vi "ZE_Recorder_CheckChannelDuplicates.vi"(8 "error in":errorcluster, 11 "Channel Array":T1 {"Terminal" items=["Default"=-1, "RSE"=10083, "NRSE"=10078, "Differential"=10106, "Pseudodifferential"=12529]}) -> (0 "error out":errorcluster, 1 "Multi Device":bool, 2 "No of channels":i16, 3 "Channel Array out":T1 caption="Channel Array" {"Terminal" items=["Default"=-1, "RSE"=10083, "NRSE"=10078, "Differential"=10106, "Pseudodifferential"=12529]})   [LabVIEW 2025, in "ZE_Recorder.lvlib"]
doc: "ZE_Recorder_CheckChannelDuplicates.vi\n----------------------------------------------\nChecks if all channels are valid and that no duplicates exist. Returns the number of valid channels or -1 in case of error.\n\nInputs:\n---------------------\n- error in : Cluster; \n- Channel Array : 1DArrayOfCluster; \n\nOutputs:\n---------------------\n- error out : Cluster; \n- No of channels : I16; \n\n----------------------------------------------\n24.08.2016\nZühlke Engineering AG\nCH-8952 Schlieren\nwww.zuehlke.com"
uses:
  ZE_Recorder.lvlib
  ZE_Recorder_ChannelCluster.ctl
  ChannelCluster.ctl
  ZE_Recorder_Units.ctl
  Temperature.ctl
panel:
  # "Connector Pane"
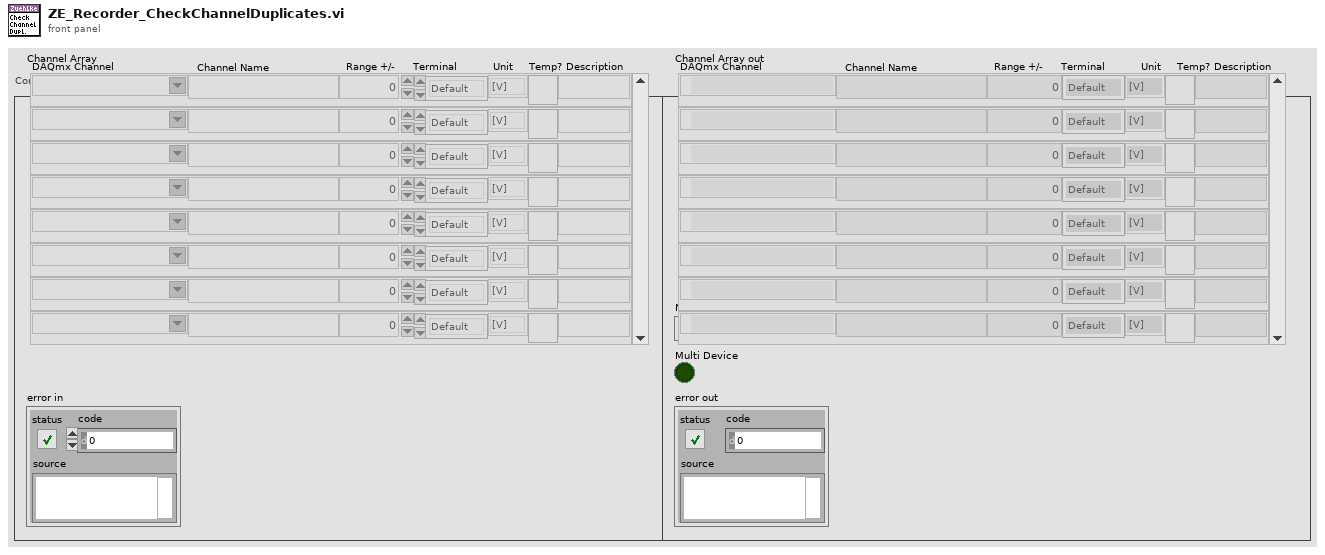
[diagram p1: front panel]
types:
  T1 = typedef "ZE_Recorder.lvlib/ZE_Recorder_ChannelCluster.ctl" = T2[]
  T2 = typedef "ZE_Recorder.lvlib/ChannelCluster.ctl" = cluster{"physical channel":tag, "channel name":string, "Range":dbl, "Terminal":i32, "Unit":T3, "isTemp":T4, "Description":string}
  T3 = typedef "ZE_Recorder.lvlib/ZE_Recorder_Units.ctl" = enum16{"[V]", "[A]", "[F]", "[H]", "[°C]", "[ml/s]", "[m/s]", "[bar]", "[%]", "[N]", "[?]"}
  T4 = typedef "ZE_Recorder.lvlib/Temperature.ctl" = bool
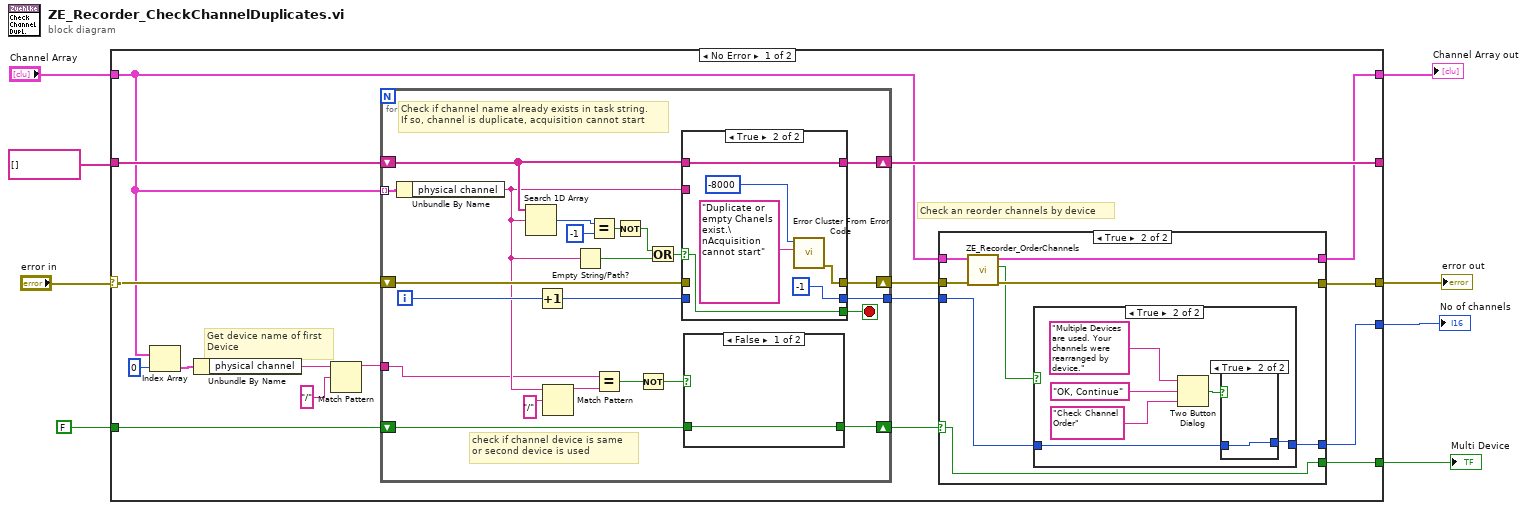
[diagram p0: block diagram]
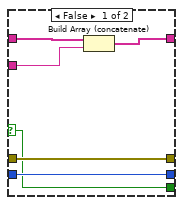
[diagram p3: hidden frame]
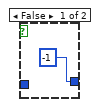
[diagram p6: hidden frame]
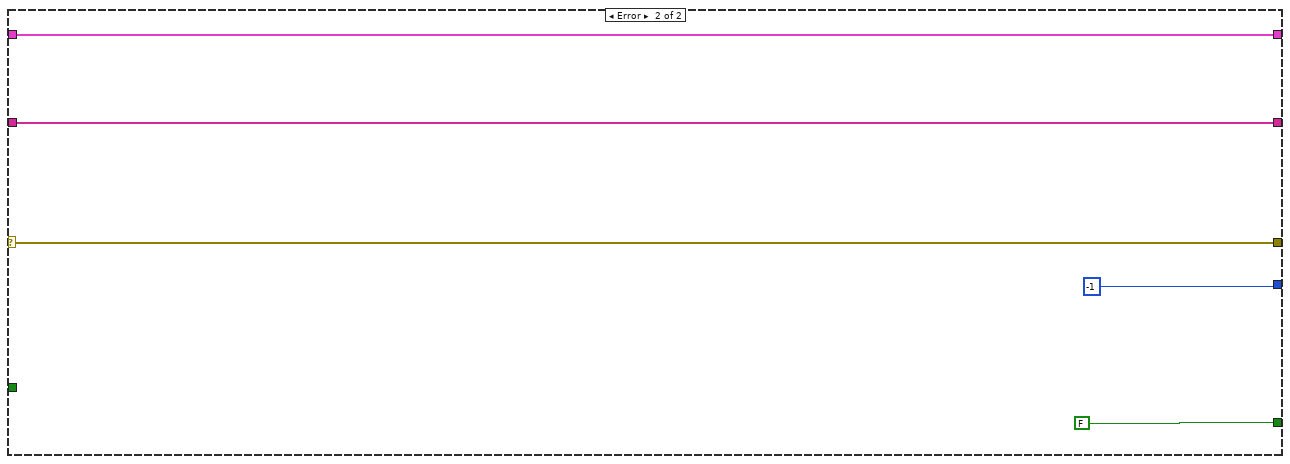
[diagram p7: hidden frame]
diagram:
  n1 = case shown="No Error" "error in" {
    selector: "error in" -> [w24 w88]
    tunnel: tag[] [] -> [w25 w87]
    tunnel: "Channel Array" -> [w13 w85]
    tunnel: [w10 w88] -> w6
    tunnel: [w23 w87] -> _
    tunnel: [w14 -1] -> w5
    tunnel: [w11 w85] -> w4
    tunnel: FALSE -> [w22 _]
    tunnel: [w9 FALSE] -> w1
    frame No Error {
      # "Check an reorder channels by device"
      # "Get device name of first\nDevice"
      n2 = Index Array(array=w13, index=0) -> (element=w20:T2)
      n3 = Unbundle By Name(w20) -> ("physical channel"=w18:tag)
      n4 = Match Pattern(string=w18, regular expression="/") -> (before substring=w17:string)  [unwired: 1 in, 3 out]
      n5 = for {
        tunnel: w13 -> [w48] mode=indexing
        shift-right: [w36] -> w23
        shift-left: w25 -> [w37]
        shift-right: [w27] -> w12
        shift-left: w24 -> [w46]
        tunnel: [w45] -> w16
        shift-right: [w28] -> w15
        shift-left: w22 -> [w30]
        tunnel: w17 -> [w29]
        i -> [w44]
        stop <- w26 stop-if-true
        # "check if channel device is same\nor second device is used"
        # "Check if channel name already exists in task string.\nIf so, channel is duplicate, acquisition cannot start"
        n6 = Unbundle By Name(w48) -> ("physical channel"=w32:tag)
        n7 = Search 1D Array(1D array=w37, element=w32) -> (index of element=w38:i32)  [unwired: 1 in]
        n8 = Increment(x=w44) -> (x+1=w43:i32)
        n9 = Match Pattern(string=w32, regular expression="/") -> (before substring=w31:string)  [unwired: 1 in, 3 out]
        n10 = Empty String/Path?(string/path=w32) -> (empty?=w39:bool)
        n11 = Equal?(x=w38, y=-1) -> (x = y?=w41:bool)
        n12 = Equal?(x=w29, y=w31) -> (x = y?=w35:bool)
        n13 = Not(x=w41) -> (.not. x?=w40:bool)
        n14 = Not(x=w35) -> (.not. x?=w34:bool)
        n15 = Or(x=w40, y=w39) -> (x .or. y?=w42:bool)
        n16 = case shown="True" w42 {
          selector: w42 -> [w54 w58]
          tunnel: w32 -> [w52 _]
          tunnel: [w56 w62] -> w27
          tunnel: w46 -> [w56 _]
          tunnel: w43 -> [w55 _]
          tunnel: [w55 -1] -> w45
          tunnel: [w54 w58] -> w26
          tunnel: w37 -> [w53 w57]
          tunnel: [w51 w57] -> w36
          frame False {
            n17 = Build Array (concatenate)(w53, w52) -> (w51:tag[])
          }
          frame True {
            n18 = call <vilib>:"Error Cluster From Error Code.vi"("error message (\"\")"="Duplicate or empty Chanels exist.\nAcquisition cannot start" ("error message (\"\")"), "error code (0)"=-8000) -> ("error out"=w62:errorcluster)  [unwired: 7 in]
          }
        }
        n19 = case shown="False" w34 {
          selector: w34 -> [_ w50]
          tunnel: w30 -> [w49 _]
          tunnel: [w49 w50] -> w28
          frame False {
          }
          frame True {
          }
        }
      }
      n20 = case shown="True" w15 {
        selector: w15 -> [w63 w67]
        tunnel: w16 -> [w66 w74]
        tunnel: [w66 w73] -> w14
        tunnel: w13 -> [w64 w72]
        tunnel: w12 -> [w65 w71]
        tunnel: [w64 w70] -> w11
        tunnel: [w65 w69] -> w10
        tunnel: [w63 w67] -> w9
        frame False {
        }
        frame True {
          n21 = call "ZE_Recorder_OrderChannels.vi"("error in"=w71, "Channel Array In"=w72) -> ("error out"=w69:errorcluster, "channels rearranged"=w68:bool, "Channel Array Out"=w70:T1)  [unwired: 7 in]
          n22 = case shown="True" w68 {
            tunnel: w74 -> [w75 w77]
            tunnel: [w75 w76] -> w73
            frame False {
            }
            frame True {
              n23 = Two Button Dialog(message="Multiple Devices are used. Your channels were rearranged by device." ("error message (\"\")"), 1:"Check Channel Order" ("F button name (\"Cancel\")"), 2:"OK, Continue" ("T button name (\"OK\")")) -> (T button?=w78:bool)
              n24 = case shown="True" w78 {
                tunnel: w77 -> [_ w83]
                tunnel: [i16 -1 ("No of channels") w83] -> w76
                frame False {
                }
                frame True {
                }
              }
            }
          }
        }
      }
    }
    frame Error {
    }
  }
  "error out" <- w6
  "No of channels" <- w5
  "Channel Array out" <- w4
  "Multi Device" <- w1
